vi "Digital Out Test_TS_v2.vi"(8 "error in":errorcluster, 11 "ControlBoard VISA":refnum<visa-resource-name>="ControlBoard") -> (0 "error out":errorcluster, 2 "Message OUT":string, 3 "Result (bool)":bool)   [LabVIEW 2022 SP3]
uses:
  <vilib>/DAQmx/read.llb/DAQmx Read (Digital 1D Bool NChan 1Samp 1Line).vi
  <vilib>/DAQmx/miscellaneous.llb/DAQmx Fill In Error Info.vi
panel:
  in  "Message IN":string
  out "Result (color)":u32(colorbox)
  out "cDAQ DI Reading":bool[](array[boolean])
  out "LC DO Cmd":bool[](array[boolean])
  out "ControlBoard VISA Out":refnum<visa-resource-name>
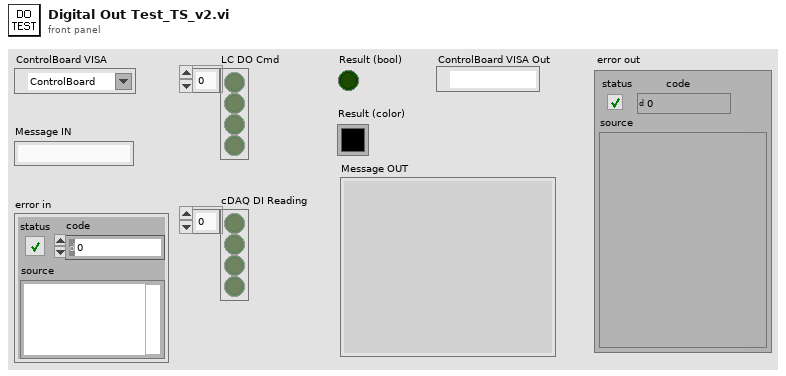
[diagram p1: front panel]
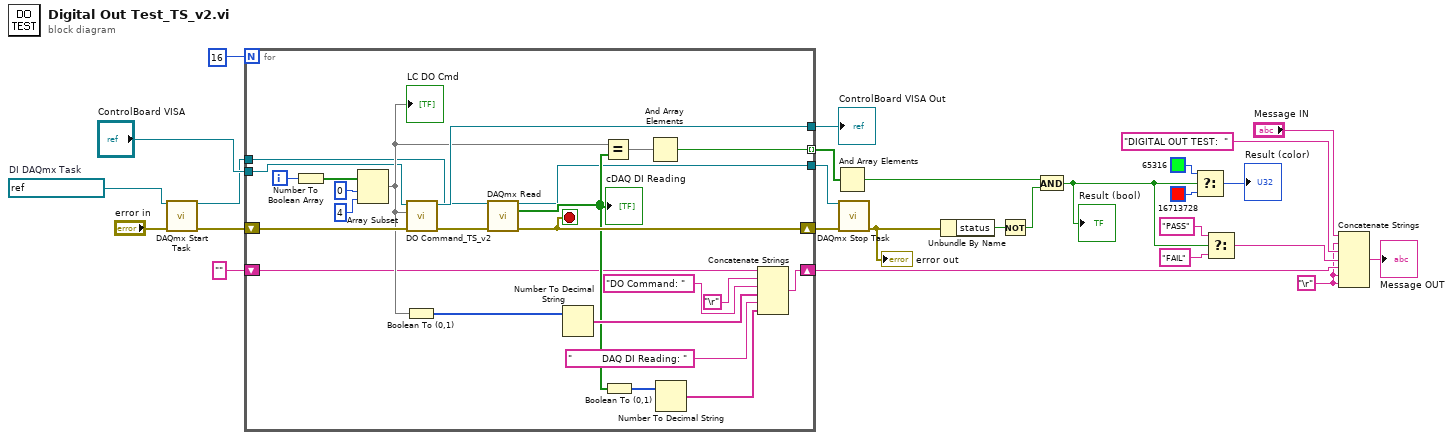
[diagram p0: block diagram]
diagram:
  w7 = refnum<k21> "BTS_DigitalIn"  # DI DAQmx Task
  w11 = "\r"
  n1 = call <vilib>:"DAQmx Start Task.vi"("task/channels in"=w7, "error in"="error in") -> ("task out"=w5:refnum<k21>, "error out"=w4:errorcluster)  [unwired: 12 in]
  n2 = for {
    N: 16 -> [_]
    shift-right: [w47] -> w1
    shift-left: w4 -> [w49]
    tunnel: [w48] -> w9
    tunnel: [w51] -> w27 mode=indexing
    shift-right: [w34] -> w16
    shift-left: "" -> [w33]
    tunnel: "ControlBoard VISA" -> [w30]
    tunnel: w5 -> [w29]
    tunnel: [w28] -> w3
    i -> [w32]
    stop <- w47 stop-if-true
    n3 = Number To Boolean Array(number=w32) -> (Boolean array=w44:bool[])
    n4 = Array Subset(array=w44, index=0, length=4) -> (w36:bool[])
    "LC DO Cmd" <- w36
    n5 = Boolean To (0,1)(Boolean=w36) -> (0, 1=w38:i16[])
    n6 = call "DO Command_TS_v2.vi"("error in (no error)"=w49, "DO Command"=w36, "ControlBoard VISA"=w30) -> ("error out"=w31:errorcluster, "ControlBoard VISA Out"=w48:refnum<visa-resource-name>)  [unwired: 7 in]
    n7 = call-poly <vilib>:"DAQmx Read.vi"("task/channels in"=w29, "error in"=w31) -> ("task out"=w28:refnum<k21>, "data"=w35:bool[], "error out"=w47:errorcluster)  [unwired: 11 in]
    "cDAQ DI Reading" <- w35
    n8 = Number To Decimal String(number=w38) -> (decimal integer string=w41:string[])  [unwired: 1 in]
    n9 = Equal?(x=w36, y=w35) -> (x = y?=w50:bool[])
    n10 = Boolean To (0,1)(Boolean=w35) -> (0, 1=w37:i16[])
    n11 = And Array Elements(Boolean array=w50) -> (logical AND=w51:bool)
    n12 = Number To Decimal String(number=w37) -> (decimal integer string=w43:string[])  [unwired: 1 in]
    n13 = Concatenate Strings(w33, "\r", "DO Command: ", w41, "          DAQ DI Reading: ", w43) -> (w34:string)
  }
  "ControlBoard VISA Out" <- w9
  n14 = And Array Elements(Boolean array=w27) -> (logical AND=w17:bool)
  n15 = call <vilib>:"DAQmx Stop Task.vi"("task/channels in"=w3, "error in"=w1) -> ("error out"=w2:errorcluster)  [unwired: 12 in, 1 out]
  "error out" <- w2
  n16 = Unbundle By Name(w2) -> ("status"=w20:bool)
  n17 = Not(x=w20) -> (.not. x?=w19:bool)
  n18 = And(x=w17, y=w19) -> (x .and. y?=w18:bool)
  "Result (bool)" <- w18
  n19 = Select(t=u32 65316 ("Result (color)"), s=w18, f=u32 16713728 ("Result (color)")) -> (s? t:f=→"Result (color)":u32)
  n20 = Select(t="PASS", s=w18, f="FAIL") -> (s? t:f=w14:string)
  n21 = Concatenate Strings("Message IN", w11, "DIGITAL OUT TEST:  ", w14, w16, w11, w11) -> (→"Message OUT":string)
